vi "FctioTest.vi"(6 "Resp Timeout":i32, 7 "Active Dut":T1, 8 "error in":errorcluster, 9 "Invert Switch":bool, 10 "FPGA Reference In":refnum<k20>, 11 "GPIO Task":refnum<k21>) -> (0 "error out":errorcluster, 2 "GPIO Outputs":string, 3 "Test Pass":bool, 5 "Elements Remaining":u32)   [LabVIEW 2018]
uses:
  Resources_Test/UART/ControlTestSlot.ctl
  <vilib>/DAQmx/read.llb/DAQmx Read (Digital 1D Bool 1Chan 1Samp).vi
  <vilib>/DAQmx/miscellaneous.llb/DAQmx Fill In Error Info.vi
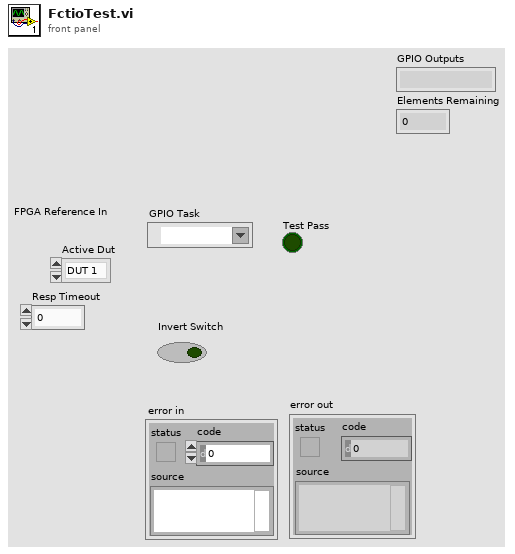
[diagram p1: front panel]
types:
  T1 = typedef "ControlTestSlot.ctl" = enum16{"DUT 1", "DUT 2"}
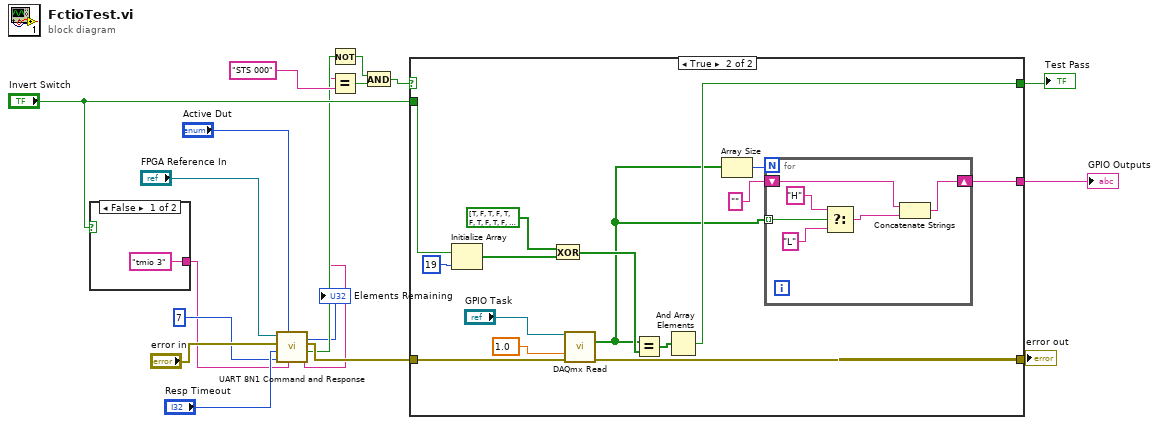
[diagram p0: block diagram]
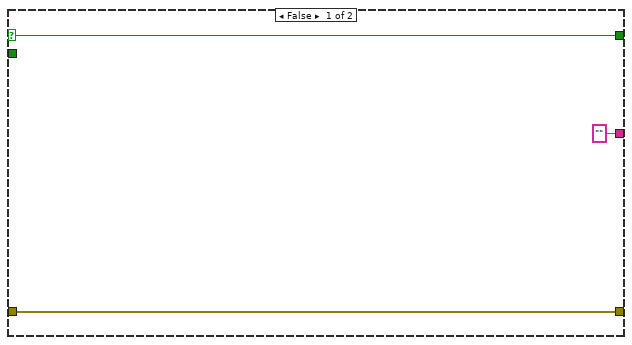
[diagram p2: hidden frame]
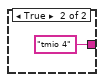
[diagram p3: hidden frame]
diagram:
  n1 = case shown="False" "Invert Switch" {
    tunnel: ["tmio 3" ("Text to Send") "tmio 4" ("Text to Send")] -> w8
    frame False {
    }
    frame True {
    }
  }
  n2 = call "UART 8N1 Command and Response.vi"("Text to Send"=w8, "Active Dut"="Active Dut", "Response Size (char)"=u32 7, "Response Timeout (ms)"="Resp Timeout", "Error In"="error in", "FPGA VI Reference In"="FPGA Reference In") -> ("Received Text"=w5:string, "Timeout Flag"=w6:bool, "Error Out"=w7:errorcluster, "Elements Remaining"=→"Elements Remaining":u32)  [unwired: 1 in, 1 out]
  n3 = Not(x=w6) -> (.not. x?=w13:bool)
  n4 = Equal?(x=w5, y="STS 000") -> (x = y?=w12:bool)
  n5 = And(x=w13, y=w12) -> (x .and. y?=w4:bool)
  n6 = case shown="True" w4 {
    selector: w4 -> [w23 _]
    tunnel: "Invert Switch" -> [_ w30]
    tunnel: [w22 w33] -> w15
    tunnel: w7 -> [w22 w32]
    tunnel: [w23 w35] -> w3
    tunnel: ["" w24] -> w2
    frame False {
    }
    frame True {
      n7 = Initialize Array(w30, 19 ("dimension size")) -> (w28:bool[])
      n8 = Exclusive Or(1:w28, 2:bool[] [TRUE, FALSE, TRUE, FALSE, TRUE, FALSE, TRUE, FALSE, TRUE, FALSE, TRUE, FALSE, TRUE, FALSE, TRUE, FALSE, TRUE, FALSE, TRUE] ("data")) -> (0:w37:bool[])
      n9 = call-poly <vilib>:"DAQmx Read.vi"("task/channels in"="GPIO Task", "timeout"=1.0, "error in"=w32) -> ("data"=w26:bool[], "error out"=w33:errorcluster)  [unwired: 10 in, 1 out]
      n10 = Equal?(x=w26, y=w37) -> (x = y?=w31:bool[])
      n11 = And Array Elements(Boolean array=w31) -> (logical AND=w35:bool)
      n12 = Array Size(array=w26) -> (size(s)=w27:i32)
      n13 = for {
        N: w27 -> [_]
        tunnel: w26 -> [w44] mode=indexing
        shift-right: [w39] -> w24
        shift-left: "" -> [w40]
        n14 = Select(t="H", s=w44, f="L") -> (s? t:f=w41:string)
        n15 = Concatenate Strings(w40, w41) -> (w39:string)
      }
    }
  }
  "Test Pass" <- w3
  "error out" <- w15
  "GPIO Outputs" <- w2
